vi "Queue Add Data to Queue.vi"(9 "Target Info in":dbl[][](array[numeric]), 10 "Stream Type":T1, 11 "Camera Index":i32) -> ()   [LabVIEW 2025]
uses:
  Vision Support Code/Steam Type.ctl
  <vilib>/Rock Robotics/Network Tables/NT PublishOptions.ctl
  <vilib>/Rock Robotics/Network Tables/NT Write Raw.vi
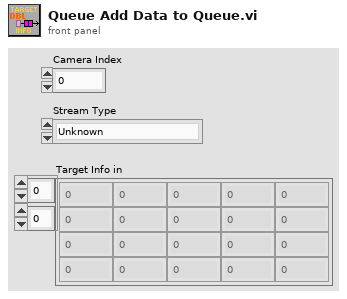
[diagram p1: front panel]
types:
  T1 = typedef "Steam Type.ctl" = enum8{"Unknown", "Apriltag", "Fuel", "Other"}
  T2 = typedef "NT PublishOptions.ctl" = cluster{"Send All":bool, "Keep Duplicates":bool, "rate (hz)":u64}
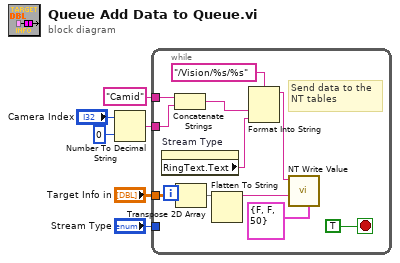
[diagram p0: block diagram]
diagram:
  n1 = Number To Decimal String(number="Camera Index", width (-)=i16 0) -> (decimal integer string=w2:string)
  n2 = while {
    tunnel: "Target Info in" -> [w17]
    tunnel: "Stream Type" -> [_]
    tunnel: "Camid" -> [w10]
    tunnel: w2 -> [w9]
    stop <- TRUE stop-if-true
    # "Send data to the NT tables"
    n3 = property on="Stream Type" class="Enum (strict)"() -> ("RingText.Text"=w7:string)  [unwired: 2 in, 2 out]
    n4 = Concatenate Strings(w10, w9) -> (w8:string)
    n5 = Transpose 2D Array(2D array=w17) -> (transposed array=w13:dbl[][])
    n6 = Flatten To String(anything=w13) -> (data string=w15:string)  [unwired: 3 in, 2 out]
    n7 = Format Into String(format string="/Vision/%s/%s", w8, w7) -> (resulting string=w11:string)  [unwired: 2 in, 1 out]
    n8 = call-poly <vilib>:"NT Write Value.vi"("options"=T2 {"Send All"=FALSE, "Keep Duplicates"=FALSE, "rate (hz)"=50}, "value"=w15, "name"=w11) -> ()  [unwired: 8 in, 1 out]
  }
